vi "tTote Autonomous.vi"   [LabVIEW 2014]
uses:
  <vilib>/Rock Robotics/WPI/RobotDrive/WPI_RobotDriveGetSetRefNum.vi
types:
  T1 = typedef "WPI_MotorControlDeviceRef.ctl" = cluster{"DeviceStatus":errorcluster, "Type":T2, "PWM":cluster{"Controller":T3, "PWM Channel":T4, "DeadBand":T5}, "CAN":cluster{"Device Number":u8, "Control Mode":T6, "Semaphore":T7, "Max Vout":dbl, "TalonSRX Control Mode":T8}, "Invert":bool, "TransformRef":T9, "InvTransformRef":T9}
  T2 = typedef "WPI_MotorControlType.ctl" = enum16{"PWM", "CAN", "CANTalonSRX"}
  T3 = typedef "FPGA_TypedefDigitalModule.ctl" = enum16{"Controller 1"}
  T4 = typedef "FPGA_DIOPWMChannel.ctl" = enum8{"PWM 0", "PWM 1", "PWM 2", "PWM 3", "PWM 4", "PWM 5", "PWM 6", "PWM 7", "PWM 8", "PWM 9", "PWM MXP 0", "PWM MXP 1", "PWM MXP 2", "PWM MXP 3", "PWM MXP 4", "PWM MXP 5", "PWM MXP 6", "PWM MXP 7", "PWM MXP 8", "PWM MXP 9", "Invalid"}
  T5 = typedef "WPI_PWMDeadband.ctl" = cluster{"Name":string, "maxPositivePwm":i32, "minPositivePwm":i32, "centerPwm":i32, "maxNegativePwm":i32, "minNegativePwm":i32, "angularRange":u16}
  T6 = typedef "WPI_CANJaguar_ControlMode.ctl" = enum8{"Percent VBus", "Current", "Speed", "Position", "Voltage"}
  T7 = typedef "Semaphore RefNum" = refnum<k1>
  T8 = typedef "WPI_CANTalonSRX_APIControlMode.ctl" = enum8{"Percent VBus", "Speed", "Position", "Slave", "Unchanged / Invalid"}
  T9 = typedef "WPI_PWMTransform_ConPane.ctl" = refnum<vi>
  T10 = typedef "WPI_EncoderDevRef.ctl" = cluster{"DevStatus":errorcluster, "EncoderIndex":T11, "CounterIndex":T12, "DistancePerCount":dbl, "Decoding Type":T13}
  T11 = typedef "FPGA_EncoderIdx.ctl" = enum8{"Enc 0", "Enc 1", "Enc 2", "Enc 3", "Enc 4", "Enc 5", "Enc 6", "Enc 7", "Invalid"}
  T12 = typedef "FPGA_CounterCtrSystemIndex.ctl" = enum8{"Ctr 0", "Ctr 1", "Ctr 2", "Ctr 3", "Ctr 4", "Ctr 5", "Ctr 6", "Ctr 7", "Invalid"}
  T13 = typedef "WPI_EncoderType.ctl" = enum16{"1x", "2x", "4x"}
  T14 = typedef "WPI_RobotDriveDevRef.ctl" = cluster{"DevStatus":errorcluster, "Motors[]":T1[], "Square Inputs":bool, "Max Output":dbl}
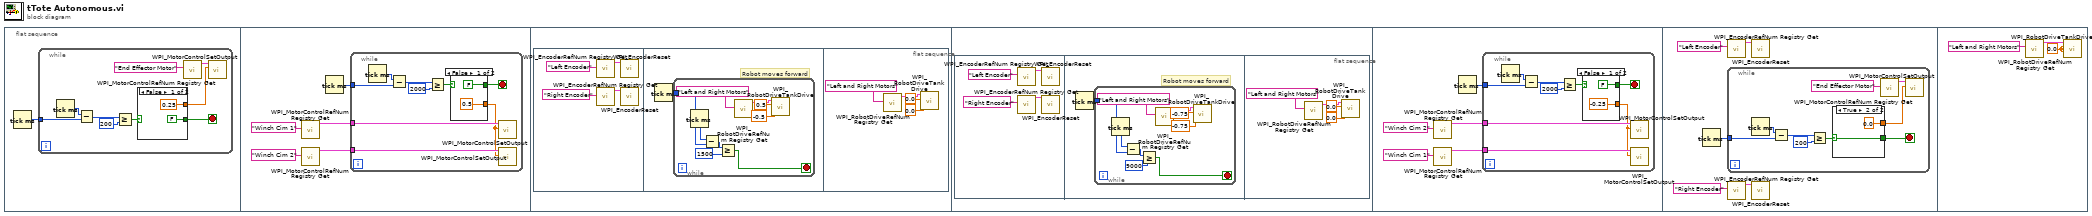
[diagram p0: block diagram]
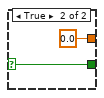
[diagram p2: hidden frame]
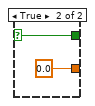
[diagram p3: hidden frame]
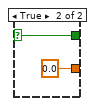
[diagram p4: hidden frame]
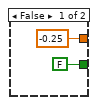
[diagram p5: hidden frame]
diagram:
  n1 = flat-sequence {
    frame #0 {
      n2 = Tick Count (ms)() -> (millisecond timer value=w1:u32)
      n3 = while {
        tunnel: w1 -> [w8]
        stop <- w3 stop-if-true
        n4 = Tick Count (ms)() -> (millisecond timer value=w9:u32)
        n5 = Subtract(x=w9, y=w8) -> (x-y=w7:u32)
        n6 = Greater Or Equal?(x=w7, y=u32 200) -> (x >= y?=w6:bool)
        n7 = case shown="False" w6 {
          selector: w6 -> [_ w13]
          tunnel: [0.25 ("Output") 0.0 ("Output")] -> w4
          tunnel: [FALSE w13] -> w3
          frame False {
          }
          frame True {
          }
        }
        n8 = call <vilib>:"WPI_MotorControlRefNum Registry Get.vi"("refnum name"="End Effector Motor") -> ("MotorControlDevRef"=w5:T1)  [unwired: 9 in, 1 out]
        n9 = call <vilib>:"WPI_MotorControlSetOutput.vi"("Output"=w4, "MotorControlDevRef"=w5) -> ()  [unwired: 7 in, 3 out]
      }
    }
    frame #1 {
      n10 = call <vilib>:"WPI_MotorControlRefNum Registry Get.vi"("refnum name"="Winch Cim 1") -> ("MotorControlDevRef"=w19:T1)  [unwired: 9 in, 1 out]
      n11 = call <vilib>:"WPI_MotorControlRefNum Registry Get.vi"("refnum name"="Winch Cim 2") -> ("MotorControlDevRef"=w16:T1)  [unwired: 9 in, 1 out]
      n12 = Tick Count (ms)() -> (millisecond timer value=w15:u32)
      n13 = while {
        tunnel: w19 -> [w24]
        tunnel: w16 -> [w23]
        tunnel: w15 -> [w25]
        stop <- w20 stop-if-true
        n14 = Tick Count (ms)() -> (millisecond timer value=w26:u32)
        n15 = Subtract(x=w26, y=w25) -> (x-y=w28:u32)
        n16 = Greater Or Equal?(x=w28, y=u32 2000) -> (x >= y?=w22:bool)
        n17 = case shown="False" w22 {
          selector: w22 -> [_ w31]
          tunnel: [0.5 ("Output") 0.0 ("Output")] -> w21
          tunnel: [FALSE w31] -> w20
          frame False {
          }
          frame True {
          }
        }
        n18 = call <vilib>:"WPI_MotorControlSetOutput.vi"("Output"=w21, "MotorControlDevRef"=w24) -> ()  [unwired: 7 in, 3 out]
        n19 = call <vilib>:"WPI_MotorControlSetOutput.vi"("Output"=w21, "MotorControlDevRef"=w23) -> ()  [unwired: 7 in, 3 out]
      }
    }
    frame #2 {
      n20 = flat-sequence {
        frame #0 {
          n21 = call <vilib>:"WPI_EncoderRefNum Registry Get.vi"("refnum name"="Left Encoder") -> ("EncoderDevRef"=w34:T10)  [unwired: 9 in, 1 out]
          n22 = call <vilib>:"WPI_EncoderRefNum Registry Get.vi"("refnum name"="Right Encoder") -> ("EncoderDevRef"=w36:T10)  [unwired: 9 in, 1 out]
          n23 = call <vilib>:"WPI_EncoderReset.vi"("EncoderDevRef"=w34) -> ()  [unwired: 9 in, 2 out]
          n24 = call <vilib>:"WPI_EncoderReset.vi"("EncoderDevRef"=w36) -> ()  [unwired: 9 in, 2 out]
        }
        frame #1 {
          # "Robot moves forward"
          n25 = Tick Count (ms)() -> (millisecond timer value=w37:u32)
          n26 = while {
            tunnel: w37 -> [w42]
            stop <- w38 stop-if-true
            n27 = Tick Count (ms)() -> (millisecond timer value=w41:u32)
            n28 = Subtract(x=w41, y=w42) -> (x-y=w40:u32)
            n29 = Greater Or Equal?(x=w40, y=u32 1500) -> (x >= y?=w38:bool)
            n30 = call <vilib>:"WPI_RobotDriveRefNum Registry Get.vi"("refnum name"="Left and Right Motors") -> ("RobotDriveDevRef"=w45:T14)  [unwired: 9 in, 1 out]
            n31 = call <vilib>:"WPI_RobotDriveTankDrive.vi"("Right axis value"=-0.5, "Left axis value"=0.5, "RobotDriveDevRef"=w45) -> ()  [unwired: 6 in, 3 out]
          }
        }
        frame #2 {
          n32 = call <vilib>:"WPI_RobotDriveRefNum Registry Get.vi"("refnum name"="Left and Right Motors") -> ("RobotDriveDevRef"=w49:T14)  [unwired: 9 in, 1 out]
          n33 = call <vilib>:"WPI_RobotDriveTankDrive.vi"("Right axis value"=0.0, "Left axis value"=0.0, "RobotDriveDevRef"=w49) -> ()  [unwired: 6 in, 3 out]
        }
      }
    }
    frame #3 {
      n34 = flat-sequence {
        frame #0 {
          n35 = call <vilib>:"WPI_EncoderRefNum Registry Get.vi"("refnum name"="Left Encoder") -> ("EncoderDevRef"=w52:T10)  [unwired: 9 in, 1 out]
          n36 = call <vilib>:"WPI_EncoderRefNum Registry Get.vi"("refnum name"="Right Encoder") -> ("EncoderDevRef"=w54:T10)  [unwired: 9 in, 1 out]
          n37 = call <vilib>:"WPI_EncoderReset.vi"("EncoderDevRef"=w52) -> ()  [unwired: 9 in, 2 out]
          n38 = call <vilib>:"WPI_EncoderReset.vi"("EncoderDevRef"=w54) -> ()  [unwired: 9 in, 2 out]
        }
        frame #1 {
          # "Robot moves forward"
          n39 = Tick Count (ms)() -> (millisecond timer value=w55:u32)
          n40 = while {
            tunnel: w55 -> [w60]
            stop <- w56 stop-if-true
            n41 = Tick Count (ms)() -> (millisecond timer value=w59:u32)
            n42 = Subtract(x=w59, y=w60) -> (x-y=w58:u32)
            n43 = Greater Or Equal?(x=w58, y=u32 9000) -> (x >= y?=w56:bool)
            n44 = call <vilib>:"WPI_RobotDriveRefNum Registry Get.vi"("refnum name"="Left and Right Motors") -> ("RobotDriveDevRef"=w63:T14)  [unwired: 9 in, 1 out]
            n45 = call <vilib>:"WPI_RobotDriveTankDrive.vi"("Right axis value"=-0.75, "Left axis value"=-0.75, "RobotDriveDevRef"=w63) -> ()  [unwired: 6 in, 3 out]
          }
        }
        frame #2 {
          n46 = call <vilib>:"WPI_RobotDriveRefNum Registry Get.vi"("refnum name"="Left and Right Motors") -> ("RobotDriveDevRef"=w67:T14)  [unwired: 9 in, 1 out]
          n47 = call <vilib>:"WPI_RobotDriveTankDrive.vi"("Right axis value"=0.0, "Left axis value"=0.0, "RobotDriveDevRef"=w67) -> ()  [unwired: 6 in, 3 out]
        }
      }
    }
    frame #4 {
      n48 = call <vilib>:"WPI_MotorControlRefNum Registry Get.vi"("refnum name"="Winch Cim 2") -> ("MotorControlDevRef"=w70:T1)  [unwired: 9 in, 1 out]
      n49 = call <vilib>:"WPI_MotorControlRefNum Registry Get.vi"("refnum name"="Winch Cim 1") -> ("MotorControlDevRef"=w73:T1)  [unwired: 9 in, 1 out]
      n50 = Tick Count (ms)() -> (millisecond timer value=w69:u32)
      n51 = while {
        tunnel: w73 -> [w78]
        tunnel: w70 -> [w77]
        tunnel: w69 -> [w79]
        stop <- w74 stop-if-true
        n52 = Tick Count (ms)() -> (millisecond timer value=w80:u32)
        n53 = Subtract(x=w80, y=w79) -> (x-y=w82:u32)
        n54 = Greater Or Equal?(x=w82, y=u32 2000) -> (x >= y?=w76:bool)
        n55 = case shown="False" w76 {
          selector: w76 -> [_ w85]
          tunnel: [-0.25 ("Output") 0.0 ("Output")] -> w75
          tunnel: [FALSE w85] -> w74
          frame False {
          }
          frame True {
          }
        }
        n56 = call <vilib>:"WPI_MotorControlSetOutput.vi"("Output"=w75, "MotorControlDevRef"=w77) -> ()  [unwired: 7 in, 3 out]
        n57 = call <vilib>:"WPI_MotorControlSetOutput.vi"("Output"=w75, "MotorControlDevRef"=w78) -> ()  [unwired: 7 in, 3 out]
      }
    }
    frame #5 {
      n58 = Tick Count (ms)() -> (millisecond timer value=w87:u32)
      n59 = call <vilib>:"WPI_EncoderRefNum Registry Get.vi"("refnum name"="Left Encoder") -> ("EncoderDevRef"=w89:T10)  [unwired: 9 in, 1 out]
      n60 = while {
        tunnel: w87 -> [w98]
        stop <- w92 stop-if-true
        n61 = Tick Count (ms)() -> (millisecond timer value=w99:u32)
        n62 = Subtract(x=w99, y=w98) -> (x-y=w97:u32)
        n63 = Greater Or Equal?(x=w97, y=u32 200) -> (x >= y?=w95:bool)
        n64 = case shown="True" w95 {
          selector: w95 -> [_ w103]
          tunnel: [-0.25 ("Output") 0.0 ("Output")] -> w93
          tunnel: [FALSE w103] -> w92
          frame False {
          }
          frame True {
          }
        }
        n65 = call <vilib>:"WPI_MotorControlRefNum Registry Get.vi"("refnum name"="End Effector Motor") -> ("MotorControlDevRef"=w94:T1)  [unwired: 9 in, 1 out]
        n66 = call <vilib>:"WPI_MotorControlSetOutput.vi"("Output"=w93, "MotorControlDevRef"=w94) -> ()  [unwired: 7 in, 3 out]
      }
      n67 = call <vilib>:"WPI_EncoderRefNum Registry Get.vi"("refnum name"="Right Encoder") -> ("EncoderDevRef"=w91:T10)  [unwired: 9 in, 1 out]
      n68 = call <vilib>:"WPI_EncoderReset.vi"("EncoderDevRef"=w89) -> ()  [unwired: 9 in, 2 out]
      n69 = call <vilib>:"WPI_EncoderReset.vi"("EncoderDevRef"=w91) -> ()  [unwired: 9 in, 2 out]
    }
    frame #6 {
      w105 = 0.0 ("Left axis value")
      n70 = call <vilib>:"WPI_RobotDriveRefNum Registry Get.vi"("refnum name"="Left and Right Motors") -> ("RobotDriveDevRef"=w106:T14)  [unwired: 9 in, 1 out]
      n71 = call <vilib>:"WPI_RobotDriveTankDrive.vi"("Right axis value"=w105, "Left axis value"=w105, "RobotDriveDevRef"=w106) -> ()  [unwired: 6 in, 3 out]
    }
  }
